vi "RefNums_Actuators.vi"() -> ()   [LabVIEW 2018]
panel:
  out "Elevator":string
  out "Drive_2R":string
  out "Drive_1R":string
  out "Upper_Intake":string
  out "Elevator_Limit_Switches":string
  out "Elevator_Brake":string
  out "Lower_Intake":string
  out "Vacuum_Pump":string
  out "PTO":string
  out "Drive_Motors":string
  out "Drive_4L":string
  out "Drive_3L":string
  out "Upper_Pulse":string
  out "Upper_Valve":string
  out "Lower_Pulse":string
  out "Lower_Valve":string
  out "Shifters":string
  out "Butterfly_Pneumatic":string
  out "Compressor":string
  out "Climber_Foot_Servo":string
  out "Hatch_Eject":string
  out "Hatch_Arm":string
  out "Spare_Victor":string
  out "Climber_Mantis":string
  out "Cargo_Arm":string
  out "Drive_System":string
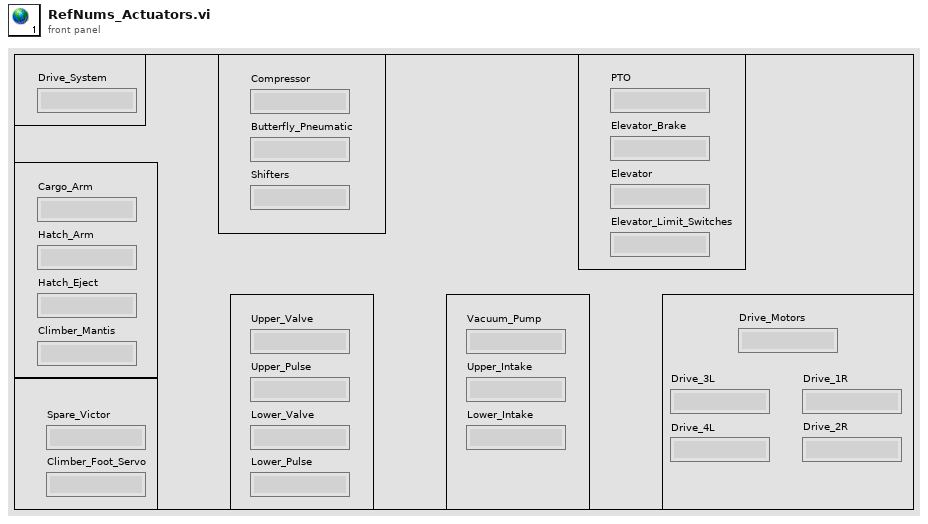
[diagram p1: front panel]
diagram:
